vi "Verify Timer.vi"(8 "error in (no error)":errorcluster, 11 "State Machine in":refnum<class "State Machine.lvclass">) -> (0 "error out":errorcluster, 2 "time out":bool, 3 "State Machine out":refnum<class "State Machine.lvclass">)   [LabVIEW 2018, in "State Machine.lvclass"]
doc: "Verify the time of the class"
uses:
  State Machine.lvclass
  State Machine.lvclass/State Machine.ctl
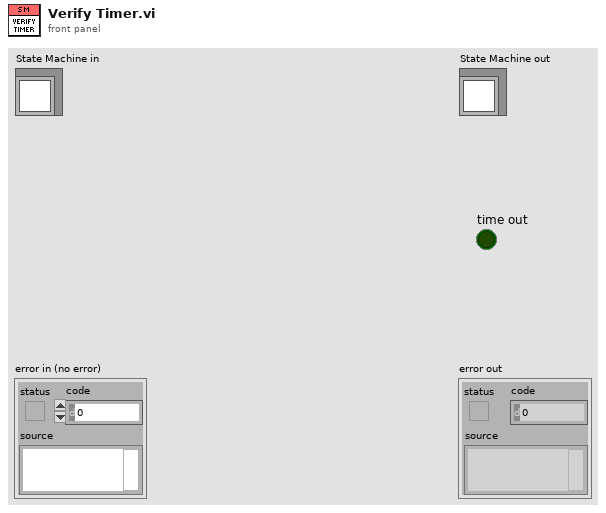
[diagram p1: front panel]
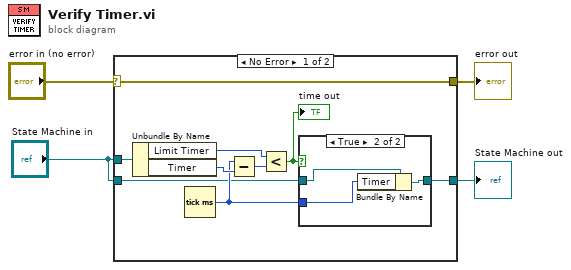
[diagram p0: block diagram]
diagram:
  n1 = case shown="No Error" "error in (no error)" {
    selector: "error in (no error)" -> [w13 w19]
    tunnel: [w13 w19] -> w3
    tunnel: [w5 w18] -> w2
    tunnel: "State Machine in" -> [w7 w18]
    tunnel: "State Machine in" -> [w6 _]
    frame No Error {
      n2 = Unbundle By Name(w7) -> ("Limit Timer"=w10:u32, "Timer"=w12:u32)
      n3 = Tick Count (ms)() -> (millisecond timer value=w8:u32)
      n4 = Subtract(x=w8, y=w12) -> (x-y=w11:u32)
      n5 = Less?(x=w10, y=w11) -> (x < y?=w9:bool)
      "time out" <- w9
      n6 = case shown="True" w9 {
        tunnel: w8 -> [_ w15]
        tunnel: w6 -> [w14 w17]
        tunnel: [w14 w16] -> w5
        frame False {
        }
        frame True {
          n7 = Bundle By Name(cluster=w17, "Timer"=w15) -> (w16:refnum<class "State Machine.lvclass">)
        }
      }
    }
    frame Error {
    }
  }
  "error out" <- w3
  "State Machine out" <- w2
